vi "Get Configuration.vi"(11 "Copy of PCAN in":refnum<class "PCAN.lvclass">) -> (2 "IConfigure":refnum<class "IStoreConfiguration.lvclass">, 3 "Copy of PCAN out":refnum<class "PCAN.lvclass">)   [LabVIEW 2024, in "PCAN.lvlib" / "PCAN.lvclass"]
uses:
  PCAN.lvclass
  PCAN.lvclass/PCAN.ctl
  Source/Interfaces/IConfigure/IStoreConfiguration.lvclass
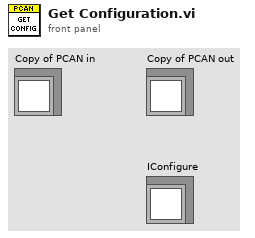
[diagram p1: front panel]
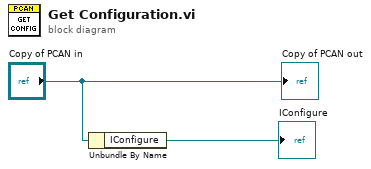
[diagram p0: block diagram]
diagram:
  n1 = Unbundle By Name("Copy of PCAN in") -> ("IConfigure"=→"IConfigure":refnum<class "IStoreConfiguration.lvclass">)
  "Copy of PCAN out" <- "Copy of PCAN in"
